vi "load regulation.vi"() -> ()   [LabVIEW 2023]
uses:
  <vilib>/Utility/file.llb/Write Delimited Spreadsheet (string).vi
panel:
  in  "Switch Button":u16(ring) items=["off", "on"]
  out "Array":dbl[](array[numeric])
  in  "error in (no error)":errorcluster
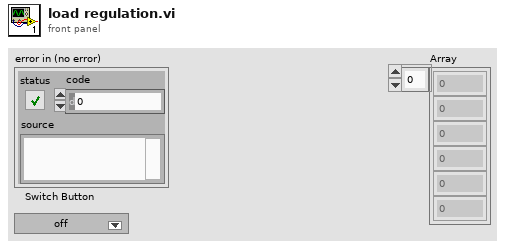
[diagram p1: front panel]
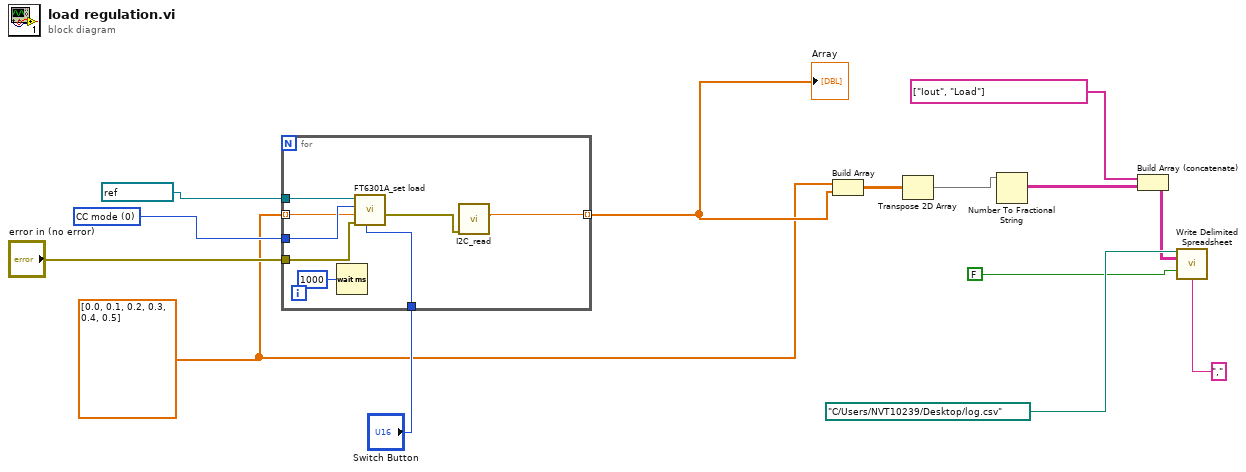
[diagram p0: block diagram]
diagram:
  w6 = dbl[] [0.0, 0.1, 0.2, 0.3, 0.4, 0.5]
  w13 = u16 0 items=["CC mode", "CR mode", "CV mode"] ("Load Mode select")
  n1 = for {
    tunnel: refnum<visa-resource-name> "FT6301A" ("VISA resource name 4") -> [w22]
    tunnel: w13 -> [w21]
    tunnel: w6 -> [w20] mode=indexing
    tunnel: "error in (no error)" -> [w17]
    tunnel: [w16] -> w7 mode=indexing
    tunnel: "Switch Button" -> [w15]
    n2 = Wait (ms)(milliseconds to wait=u32 1000) -> ()  [unwired: 1 out]
    n3 = call "FT6301A_set load.vi"("Switch Button"=w15, "error in (no error)"=w17, "Load Parameter"=w20, "Load Mode select"=w21, "VISA resource name 4"=w22) -> ("error out"=w18:errorcluster)  [unwired: 6 in]
    n4 = call "I2C_read.vi"("error in (no error)"=w18) -> ("x/y"=w16:dbl)  [unwired: 9 in, 1 out]
  }
  "Array" <- w7
  n5 = Build Array(w6, w7) -> (w5:dbl[][])
  n6 = Transpose 2D Array(2D array=w5) -> (transposed array=w4:dbl[][])
  n7 = Number To Fractional String(number=w4) -> (F-format string=w3:string[][])  [unwired: 3 in]
  n8 = Build Array (concatenate)(string[] ["Iout", "Load"], w3) -> (w1:string[][])
  n9 = call-poly <vilib>:"Write Delimited Spreadsheet.vi"("file path (dialog if empty)"=path "C:/Users/NVT10239/Desktop/log.csv" ("file path (use dialog)"), "2D data"=w1, "append to file? (new file:F)"=FALSE, "delimiter (\\t)"="," ("delimiter (\\t)")) -> ()  [unwired: 10 in, 2 out]
